vi "SaveDeviceHeader.vi"(0 "File Refnum in":refnum<file>, 5 "Filename":string, 7 "Run Number":i32, 9 "Array Titles":string, 11 "error in (no error)":errorcluster, 12 "Temperature":dbl, 13 "Humidity":dbl, 14 "Strip Structure":string) -> (4 "File Refnum out":refnum<file>, 6 "Header string":string, 10 "error out":errorcluster)   [LabVIEW 2019]
uses:
  globals/QC_RunInformation.vi
  globals/QC_MeasurementSetup.vi
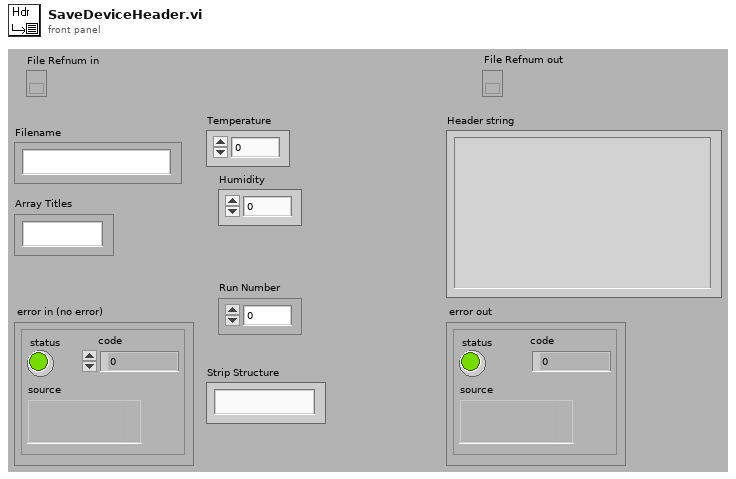
[diagram p1: front panel]
types:
  T1 = cluster{"Sensor Serial No.:":string, "Wafer Serial No.:":string, "Batch:":string, "Manufacturer:":string, "Device Category:":string, "Database Serial No.:":string, "Date Initiated:":string, "Time Initiated:":string, "Test":string, "Instruments used:":string, "Probeplan used:":string, "End of Run comment:":string, "User:":string}
  T2 = cluster{"Institute":string, "Manufacturers":string[], "Devices":string[], "Serialnumbers Lookup DB":string, "Data directory":string, "Backup & screenshot directory":string, "List of known users":string[], "Measurement switch not used":bool, "Measurement Switch":string, "DUT Switch":string}
  T3 = cluster{"Supply":refnum<class "SupplyControl.lvclass">, "LCR":refnum<class "LCRControl.lvclass">, "Initial Voltage [V]":dbl, "Final Voltage [V]":dbl, "Step Size [V]":dbl, "Step Interval [s]":i32, "Number Of Steps":u32, "AC frequency [Hz]":i32, "RC Configuration":u16, "AC amplitude [V]":dbl, "Ramp down steps [V]":dbl, "Ramp down Interval [s]":i32, "Set Current Limit?":bool, "Current Limit [µA]":dbl, "Temperature Readout":enum16{"Read Arduino", "Enter manually"}, "Arduino":refnum<class "ArduinoControl.lvclass">, "Supply Name":string, "LCR Name":string, "V_depletion Limit [V]":dbl, "Switching":refnum<class "Switching.lvclass">, "Matrix used?":bool, "Matrix X Channels":cluster{"Bias Supply / SMU LO":i32, "Bias Supply / SMU HI":i32, "CV Box LO":i32, "CV Box HI":i32, "CV Box LO IN":i32, "CV Box HI IN":i32, "Volt meter LO":i32, "Volt meter HI":i32, "Mux1 C1":i32, "Mux1 C2":i32, "Mux2 C1":i32, "Mux2 C2":i32}}
  T4 = cluster{"Bias Supply":refnum<class "SupplyControl.lvclass">, "SMU":refnum<class "SupplyControl.lvclass">, "LCR":refnum<class "LCRControl.lvclass">, "Probe Card Channels":i32, "Bias Voltage [V]":dbl, "First strip":i32, "Last strip":i32, "Base Voltage [V]":dbl, "Base Ramp Step [V]":dbl, "Base Ramp Interval [ms]":u32, "High Voltage [V]":dbl, "High Ramp Step [V]":dbl, "High Ramp Interval [ms]":u32, "AC frequency [Hz]":i32, "AC amplitude [V]":dbl, "RC Configuration":u16, "Single Needle":bool, "Temperature Readout":enum16{"Read Arduino", "Enter manually"}, "Arduino":refnum<class "ArduinoControl.lvclass">, "Fraction of good strips [%]":dbl, "ProbeStation":refnum<class "ProbeStationControl.lvclass">, "Switching":refnum<class "Switching.lvclass">, "Matrix used?":bool, "Matrix X Channels":cluster{"Bias Supply / SMU LO":i32, "Bias Supply / SMU HI":i32, "CV Box LO":i32, "CV Box HI":i32, "CV Box LO IN":i32, "CV Box HI IN":i32, "Volt meter LO":i32, "Volt meter HI":i32, "Mux1 C1":i32, "Mux1 C2":i32, "Mux2 C1":i32, "Mux2 C2":i32}, "Pinholes Y/N":bool, "Capacitance Y/N":bool, "Resistance Y/N":bool, "Bias Supply Name":string, "SMU Name":string, "LCR Name":string}
  T5 = cluster{"Supply":refnum<class "SupplyControl.lvclass">, "LCR":refnum<class "LCRControl.lvclass">, "Initial Voltage [V]":dbl, "Final Voltage [V]":dbl, "Step Size [V]":dbl, "Step Interval [s]":i32, "Number Of Steps":u32, "AC frequency [Hz]":i32, "RC Configuration":u16, "AC amplitude [V]":dbl, "Ramp down steps [V]":dbl, "Ramp down Interval [s]":i32, "Set Current Limit?":bool, "Current Limit [µA]":dbl, "Temperature Readout":enum16{"Read Arduino", "Enter manually"}, "Arduino":refnum<class "ArduinoControl.lvclass">, "Supply Name":string, "LCR Name":string, "C_is Limit [pF/cm]":dbl, "Switching":refnum<class "Switching.lvclass">, "Matrix used?":bool, "Matrix X Channels":cluster{"Bias Supply / SMU LO":i32, "Bias Supply / SMU HI":i32, "CV Box LO":i32, "CV Box HI":i32, "CV Box LO IN":i32, "CV Box HI IN":i32, "Volt meter LO":i32, "Volt meter HI":i32, "Mux1 C1":i32, "Mux1 C2":i32, "Mux2 C1":i32, "Mux2 C2":i32}, "Structure Name":string}
  T6 = cluster{"Bias Supply":refnum<class "SupplyControl.lvclass">, "SMU":refnum<class "SupplyControl.lvclass">, "Multimeter":refnum<class "MultimeterControl.lvclass">, "Initial Voltage [V]":dbl, "Final Voltage [V]":dbl, "Step Size [V]":dbl, "Step Interval [s]":i32, "Number Of Steps":u32, "Ramp down steps [V]":dbl, "Ramp down Interval [s]":i32, "Set Current Limit?":bool, "Current Limit [µA]":dbl, "Temperature Readout":enum16{"Read Arduino", "Enter manually"}, "Arduino":refnum<class "ArduinoControl.lvclass">, "Supply Name":string, "SMU Name":string, "Voltmeter Name":string, "R_is Limit [MOhm]":dbl, "Switching":refnum<class "Switching.lvclass">, "Matrix used?":bool, "Matrix X Channels":cluster{"Bias Supply / SMU LO":i32, "Bias Supply / SMU HI":i32, "CV Box LO":i32, "CV Box HI":i32, "CV Box LO IN":i32, "CV Box HI IN":i32, "Volt meter LO":i32, "Volt meter HI":i32, "Mux1 C1":i32, "Mux1 C2":i32, "Mux2 C1":i32, "Mux2 C2":i32}, "Structure Name":string}
  T7 = cluster{"Supply":refnum<class "SupplyControl.lvclass">, "Final Test Voltage [V]":dbl, "Bias Voltage [V]":dbl, "Bias Step Size [V]":dbl, "Step Interval [s]":i32, "Bias Number of Steps":u32, "Ramp down steps [V]":dbl, "Ramp down Interval [s]":i32, "Set Current Limit?":bool, "Current Limit Bias [µA]":dbl, "Temperature Readout":enum16{"Read Arduino", "Enter manually"}, "Arduino":refnum<class "ArduinoControl.lvclass">, "Supply Name":string, "V_breakdown Limit [V]":dbl, "Switching":refnum<class "Switching.lvclass">, "Matrix used?":bool, "Matrix X Channels":cluster{"Bias Supply / SMU LO":i32, "Bias Supply / SMU HI":i32, "CV Box LO":i32, "CV Box HI":i32, "CV Box LO IN":i32, "CV Box HI IN":i32, "Volt meter LO":i32, "Volt meter HI":i32, "Mux1 C1":i32, "Mux1 C2":i32, "Mux2 C1":i32, "Mux2 C2":i32}, "SMU Name":string, "Test Step Size [V] ":dbl, "Test Number of Steps ":u32, "SMU":refnum<class "SupplyControl.lvclass">, "Current Limit SMU [µA] ":dbl, "Structure Name":string}
  T8 = cluster{"Supply":refnum<class "SupplyControl.lvclass">, "Initial Voltage [V]":dbl, "Final Voltage [V]":dbl, "Step Size [V]":dbl, "Step Interval [s]":i32, "Number Of Steps":u32, "Ramp down steps [V]":dbl, "Ramp down Interval [s]":i32, "Set Current Limit?":bool, "Current Limit [µA]":dbl, "Temperature Readout":enum16{"Read Arduino", "Enter manually"}, "Arduino":refnum<class "ArduinoControl.lvclass">, "Supply Name":string, "Switching":refnum<class "Switching.lvclass">, "Matrix used?":bool, "Matrix X Channels":cluster{"Bias Supply / SMU LO":i32, "Bias Supply / SMU HI":i32, "CV Box LO":i32, "CV Box HI":i32, "CV Box LO IN":i32, "CV Box HI IN":i32, "Volt meter LO":i32, "Volt meter HI":i32, "Mux1 C1":i32, "Mux1 C2":i32, "Mux2 C1":i32, "Mux2 C2":i32}, "Structure Name":string}
  T9 = cluster{"Supply":refnum<class "SupplyControl.lvclass">, "Initial Current [uA]":dbl, "Final Current [uA]":dbl, "Step Size [uA]":dbl, "Step Interval [s]":i32, "Number Of Steps":u32, "Ramp down steps [uA]":dbl, "Ramp down Interval [s]":i32, "Set Current Limit?":bool, "Voltage Limit [mV]":dbl, "Temperature Readout":enum16{"Read Arduino", "Enter manually"}, "Arduino":refnum<class "ArduinoControl.lvclass">, "Supply Name":string, "Switching":refnum<class "Switching.lvclass">, "Matrix used?":bool, "Matrix X Channels":cluster{"Bias Supply / SMU LO":i32, "Bias Supply / SMU HI":i32, "CV Box LO":i32, "CV Box HI":i32, "CV Box LO IN":i32, "CV Box HI IN":i32, "Volt meter LO":i32, "Volt meter HI":i32, "Mux1 C1":i32, "Mux1 C2":i32, "Mux2 C1":i32, "Mux2 C2":i32}, "Structure Name":string}
  T10 = cluster{"Supply":refnum<class "SupplyControl.lvclass">, "LCR":refnum<class "LCRControl.lvclass">, "Initial Voltage [V]":dbl, "Final Voltage [V]":dbl, "Step Size [V]":dbl, "Step Interval [s]":i32, "Number Of Steps":u32, "AC frequency [Hz]":i32, "RC Configuration":u16, "AC amplitude [V]":dbl, "Ramp down steps [V]":dbl, "Ramp down Interval [s]":i32, "Set Current Limit?":bool, "Current Limit [µA]":dbl, "Temperature Readout":enum16{"Read Arduino", "Enter manually"}, "Arduino":refnum<class "ArduinoControl.lvclass">, "Supply Name":string, "LCR Name":string, "V_depletion Limit [V]":dbl, "Switching":refnum<class "Switching.lvclass">, "Matrix used?":bool, "Matrix X Channels":cluster{"Bias Supply / SMU LO":i32, "Bias Supply / SMU HI":i32, "CV Box LO":i32, "CV Box HI":i32, "CV Box LO IN":i32, "CV Box HI IN":i32, "Volt meter LO":i32, "Volt meter HI":i32, "Mux1 C1":i32, "Mux1 C2":i32, "Mux2 C1":i32, "Mux2 C2":i32}, "Structure Name":string}
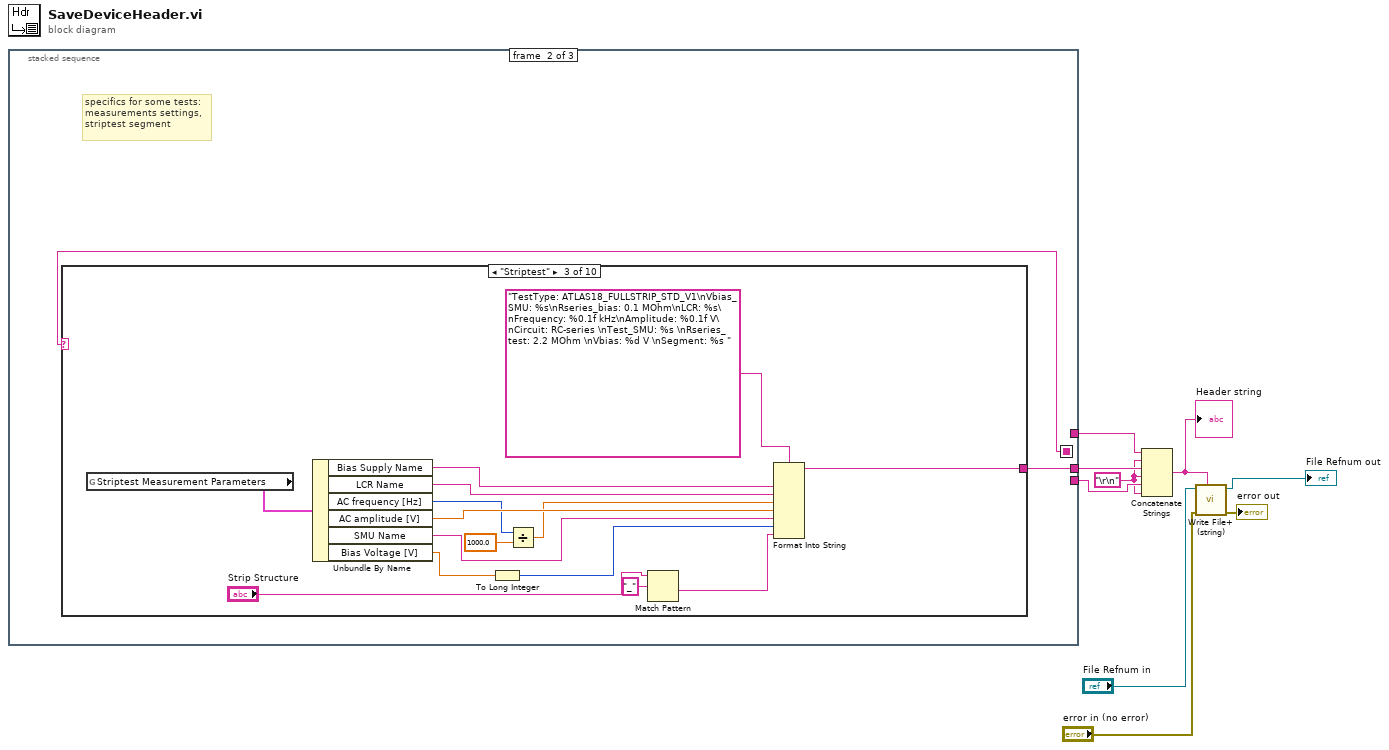
[diagram p0: block diagram]
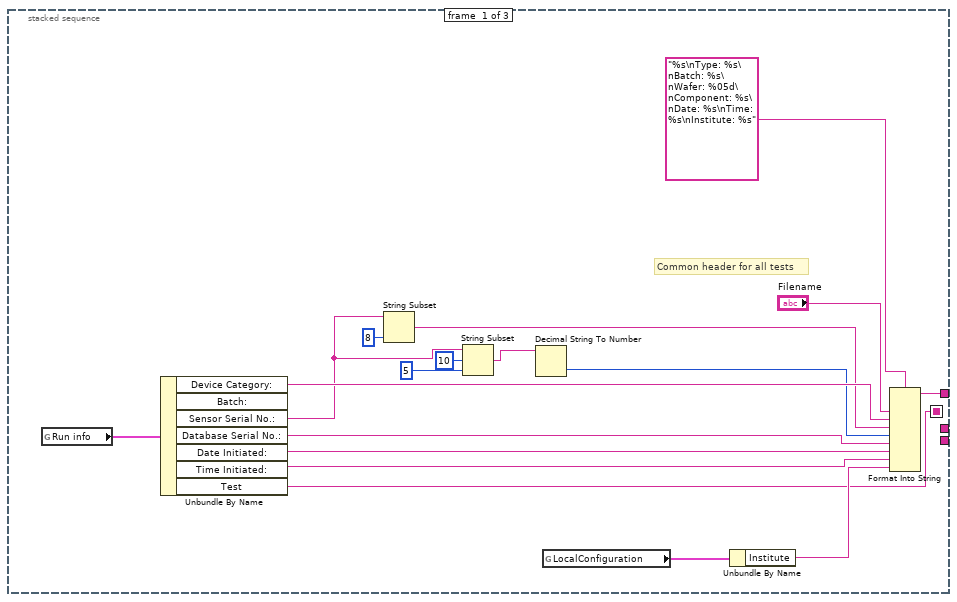
[diagram p2: hidden frame]
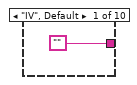
[diagram p3: hidden frame]
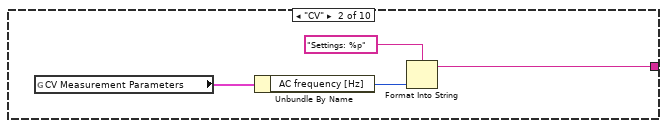
[diagram p4: hidden frame]
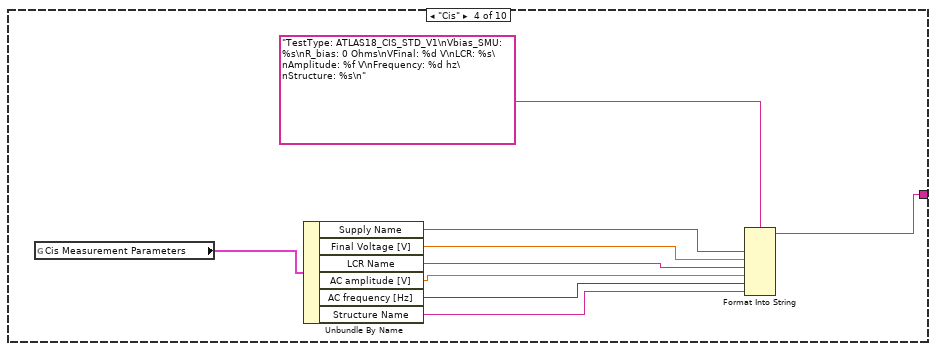
[diagram p5: hidden frame]
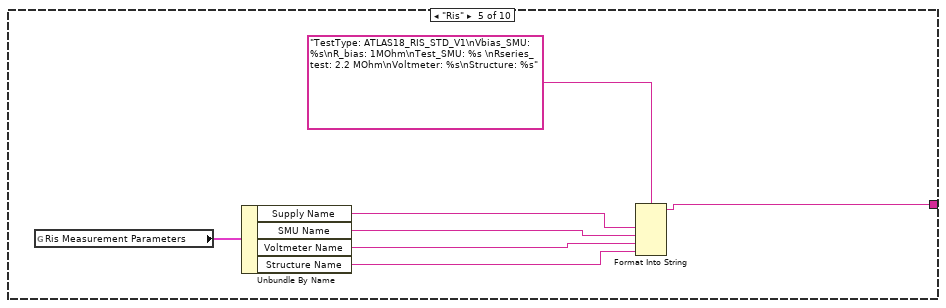
[diagram p6: hidden frame]
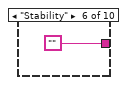
[diagram p7: hidden frame]
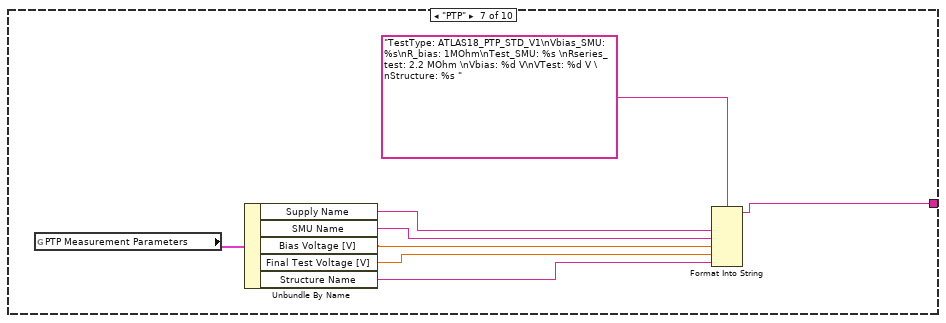
[diagram p8: hidden frame]
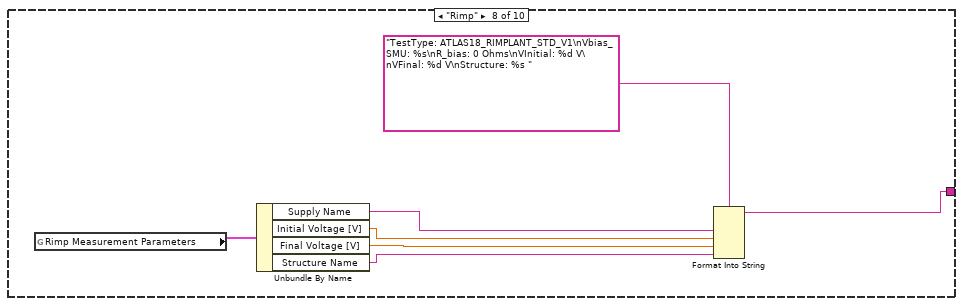
[diagram p9: hidden frame]
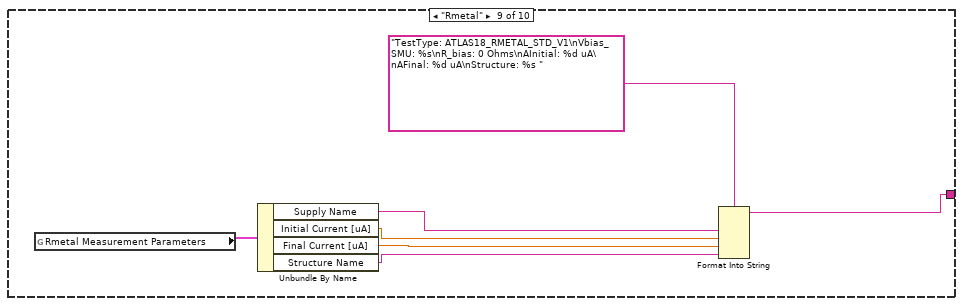
[diagram p10: hidden frame]
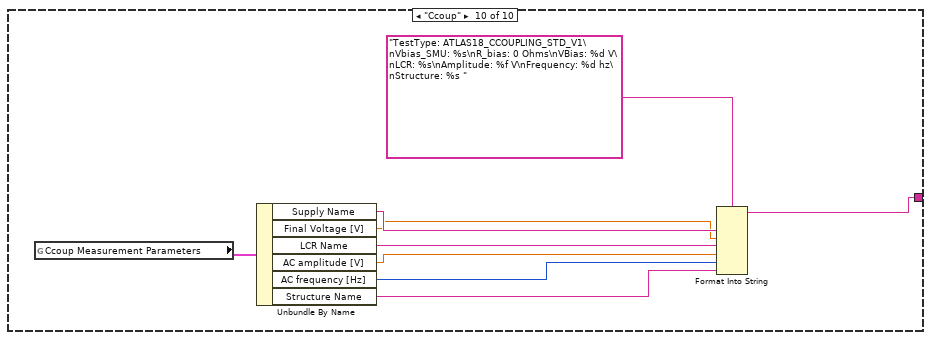
[diagram p11: hidden frame]
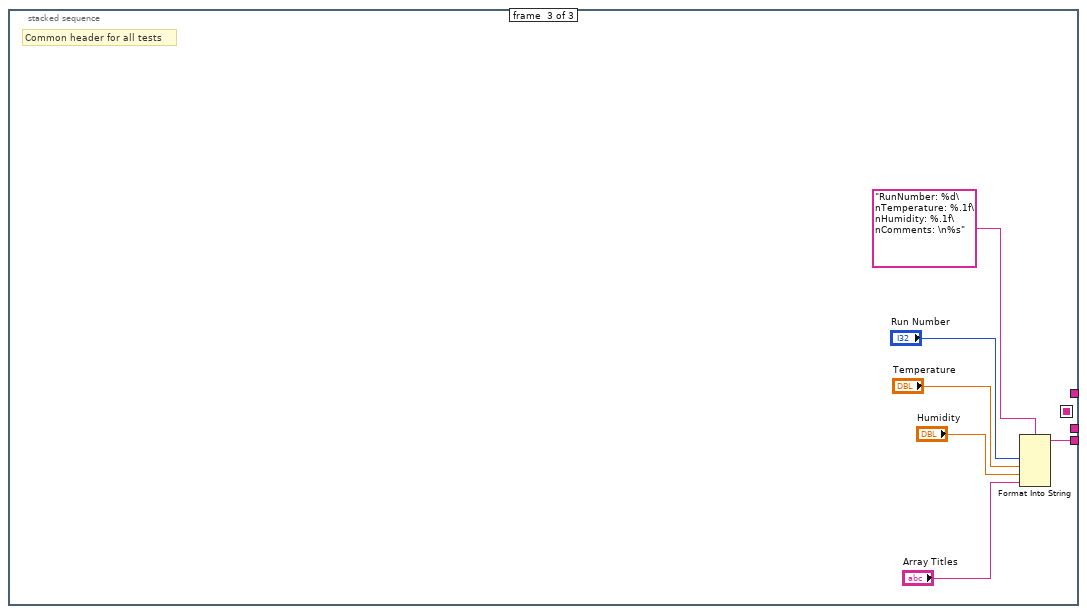
[diagram p12: hidden frame]
diagram:
  w1 = "\r\n"
  n1 = stacked-sequence {
    seq-local: [w17 _ _] -> [_ w29 _]
    tunnel: [_ w28 _] -> w5
    tunnel: [_ _ w99] -> w4
    tunnel: [w23 _ _] -> w3
    frame #0 {
      # "Common header for all tests"
      n2 = global read "QC_RunInformation.vi" "Run info"() -> (w25:T1)
      n3 = Unbundle By Name(w25) -> ("Device Category:"=w22:string, "Sensor Serial No.:"=w14:string, "Database Serial No.:"=w21:string, "Date Initiated:"=w20:string, "Time Initiated:"=w19:string, "Test"=w17:string)  [unwired: 1 out]
      n4 = String Subset(string=w14, length (rest)=8 ("length (rest)")) -> (substring=w15:string)  [unwired: 1 in]
      n5 = String Subset(string=w14, offset (0)=10, length (rest)=5 ("length (rest)")) -> (substring=w11:string)
      n6 = Decimal String To Number(string=w11) -> (number=w10:i32)  [unwired: 2 in, 1 out]
      n7 = global read "QC_RunInformation.vi" "LocalConfiguration"() -> (w24:T2)
      n8 = Unbundle By Name(w24) -> ("Institute"=w18:string)
      n9 = Format Into String(format string="%s\nType: %s\nBatch: %s\nWafer: %05d\nComponent: %s\nDate: %s\nTime: %s\nInstitute: %s", "Filename", w22, w15, w10, w21, w20, w19, w18) -> (resulting string=w23:string)  [unwired: 2 in, 1 out]
    }
    frame #1 {
      # "specifics for some tests:\nmeasurements settings,\nstriptest segment"
      n10 = case shown="\"Striptest\"" w29 {
        tunnel: ["" w31 w47 w51 w60 "" w68 w75 w82 w89] -> w28
        frame "IV", Default {
        }
        frame "CV" {
          n11 = global read "QC_MeasurementSetup.vi" "CV Measurement Parameters"() -> (w32:T3)
          n12 = Unbundle By Name(w32) -> ("AC frequency [Hz]"=w34:i32)
          n13 = Format Into String(format string="Settings: %p", w34) -> (resulting string=w31:string)  [unwired: 2 in, 1 out]
        }
        frame "Striptest" {
          n14 = global read "QC_MeasurementSetup.vi" "Striptest Measurement Parameters"() -> (w49:T4)
          n15 = Unbundle By Name(w49) -> ("Bias Supply Name"=w46:string, "LCR Name"=w45:string, "AC frequency [Hz]"=w42:i32, "AC amplitude [V]"=w44:dbl, "SMU Name"=w40:string, "Bias Voltage [V]"=w39:dbl)
          n16 = To Long Integer(number=w39) -> (32bit integer=w38:i32)
          n17 = Divide(x=w42, y=1000.0) -> (x/y=w41:dbl)
          n18 = Match Pattern(string="Strip Structure", regular expression="_") -> (after substring=w35:string)  [unwired: 1 in, 3 out]
          n19 = Format Into String(format string="TestType: ATLAS18_FULLSTRIP_STD_V1\nVbias_SMU: %s\nRseries_bias: 0.1 MOhm\nLCR: %s\nFrequency: %0.1f kHz\nAmplitude: %0.1f V\nCircuit: RC-series \nTest_SMU: %s \nRseries_test: 2.2 MOhm \nVbias: %d V \nSegment: %s ", w46, w45, w41, w44, w40, w38, w35) -> (resulting string=w47:string)  [unwired: 2 in, 1 out]
        }
        frame "Cis" {
          n20 = global read "QC_MeasurementSetup.vi" "Cis Measurement Parameters"() -> (w55:T5)
          n21 = Unbundle By Name(w55) -> ("Supply Name"=w58:string, "Final Voltage [V]"=w57:dbl, "LCR Name"=w56:string, "AC amplitude [V]"=w53:dbl, "AC frequency [Hz]"=w52:i32, "Structure Name"=w50:string)
          n22 = Format Into String(format string="TestType: ATLAS18_CIS_STD_V1\nVbias_SMU: %s\nR_bias: 0 Ohms\nVFinal: %d V\nLCR: %s\nAmplitude: %f V\nFrequency: %d hz\nStructure: %s\n", w58, w57, w56, w53, w52, w50) -> (resulting string=w51:string)  [unwired: 2 in, 1 out]
        }
        frame "Ris" {
          n23 = global read "QC_MeasurementSetup.vi" "Ris Measurement Parameters"() -> (w65:T6)
          n24 = Unbundle By Name(w65) -> ("Supply Name"=w63:string, "SMU Name"=w62:string, "Voltmeter Name"=w61:string, "Structure Name"=w59:string)
          n25 = Format Into String(format string="TestType: ATLAS18_RIS_STD_V1\nVbias_SMU: %s\nR_bias: 1MOhm\nTest_SMU: %s \nRseries_test: 2.2 MOhm\nVoltmeter: %s\nStructure: %s", w63, w62, w61, w59) -> (resulting string=w60:string)  [unwired: 2 in, 1 out]
        }
        frame "Stability" {
        }
        frame "PTP" {
          n26 = global read "QC_MeasurementSetup.vi" "PTP Measurement Parameters"() -> (w74:T7)
          n27 = Unbundle By Name(w74) -> ("Supply Name"=w73:string, "SMU Name"=w72:string, "Bias Voltage [V]"=w70:dbl, "Final Test Voltage [V]"=w71:dbl, "Structure Name"=w67:string)
          n28 = Format Into String(format string="TestType: ATLAS18_PTP_STD_V1\nVbias_SMU: %s\nR_bias: 1MOhm\nTest_SMU: %s \nRseries_test: 2.2 MOhm \nVbias: %d V\nVTest: %d V \nStructure: %s ", w73, w72, w70, w71, w67) -> (resulting string=w68:string)  [unwired: 2 in, 1 out]
        }
        frame "Rimp" {
          n29 = global read "QC_MeasurementSetup.vi" "Rimp Measurement Parameters"() -> (w81:T8)
          n30 = Unbundle By Name(w81) -> ("Supply Name"=w80:string, "Initial Voltage [V]"=w77:dbl, "Final Voltage [V]"=w79:dbl, "Structure Name"=w76:string)
          n31 = Format Into String(format string="TestType: ATLAS18_RIMPLANT_STD_V1\nVbias_SMU: %s\nR_bias: 0 Ohms\nVInitial: %d V\nVFinal: %d V\nStructure: %s ", w80, w77, w79, w76) -> (resulting string=w75:string)  [unwired: 2 in, 1 out]
        }
        frame "Rmetal" {
          n32 = global read "QC_MeasurementSetup.vi" "Rmetal Measurement Parameters"() -> (w88:T9)
          n33 = Unbundle By Name(w88) -> ("Supply Name"=w87:string, "Initial Current [uA]"=w84:dbl, "Final Current [uA]"=w86:dbl, "Structure Name"=w83:string)
          n34 = Format Into String(format string="TestType: ATLAS18_RMETAL_STD_V1\nVbias_SMU: %s\nR_bias: 0 Ohms\nAInitial: %d uA\nAFinal: %d uA\nStructure: %s ", w87, w84, w86, w83) -> (resulting string=w82:string)  [unwired: 2 in, 1 out]
        }
        frame "Ccoup" {
          n35 = global read "QC_MeasurementSetup.vi" "Ccoup Measurement Parameters"() -> (w97:T10)
          n36 = Unbundle By Name(w97) -> ("Supply Name"=w95:string, "Final Voltage [V]"=w94:dbl, "LCR Name"=w93:string, "AC amplitude [V]"=w92:dbl, "AC frequency [Hz]"=w91:i32, "Structure Name"=w90:string)
          n37 = Format Into String(format string="TestType: ATLAS18_CCOUPLING_STD_V1\nVbias_SMU: %s\nR_bias: 0 Ohms\nVBias: %d V\nLCR: %s\nAmplitude: %f V\nFrequency: %d hz\nStructure: %s ", w95, w94, w93, w92, w91, w90) -> (resulting string=w89:string)  [unwired: 2 in, 1 out]
        }
      }
    }
    frame #2 {
      # "Common header for all tests"
      n38 = Format Into String(format string="RunNumber: %d\nTemperature: %.1f\nHumidity: %.1f\nComments: \n%s", "Run Number", "Temperature", "Humidity", "Array Titles") -> (resulting string=w99:string)  [unwired: 2 in, 1 out]
    }
  }
  n39 = Concatenate Strings(w3, w1, w5, w1, w4, w1) -> (w2:string)
  "Header string" <- w2
  n40 = call <vilib>:"Write File+ (string).vi"("string"=w2, "error in (no error)"="error in (no error)", "refnum"="File Refnum in") -> ("error out"=→"error out":errorcluster, "dup refnum"=→"File Refnum out":refnum<file>)  [unwired: 4 in, 1 out]
